vi "Send Test.vi"() -> ()   [LabVIEW 2009]
uses:
  UDP Lib/UDP Network Location.ctl
  Support Files/Address.ctl
  <vilib>/Platform/TimedLoop/XDataNode/XDataNode.xnode
  <vilib>/Platform/TimedLoop/XDataNode/loadlvalarms.vi
  <vilib>/Platform/TimedLoop/XDataNode/timing_clust.ctl
  <vilib>/Platform/TimedLoop/XDataNode/nitl_modes.ctl
  <vilib>/Platform/TimedLoop/XDataNode/wakeup.ctl
  <vilib>/Platform/TimedLoop/XDataNode/XDNodeRunTimeDep.lvlib
panel:
  out "Network Location":T1={"IP Address"="0.0.0.0", "Port"=0}
  out "Address Cluster":T2={"Subsystem Id"=90, "Node Id"=1, "Component Id"=1}
  out "Payload":string
  out "UDP Read Loop":bool=TRUE
  out "HB":bool
  in  "stop":bool
  in  "Destination Location":T1={"IP Address"="localhost", "Port"=3794}
  in  "Send":bool
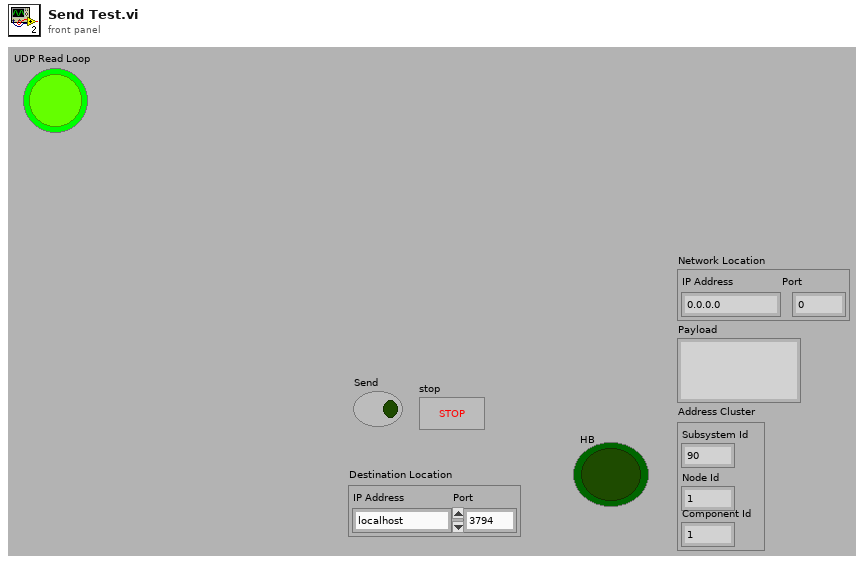
[diagram p1: front panel]
types:
  T1 = typedef "UDP Network Location.ctl" = cluster{"IP Address":string, "Port":u16}
  T2 = typedef "Address.ctl" = cluster{"Subsystem Id":u16, "Node Id":u8, "Component Id":u8}
  T3 = typedef "UDP Base.ctl" = cluster{"UDP Session":refnum<k16>, "UDP Socket Params":T4}
  T4 = typedef "UDP Socket Params.ctl" = cluster{"Local Port":u16, "Read Timeout":i32, "Write Timeout":i32}
  T5 = typedef "XDNodeRunTimeDep.lvlib/timing_clust.ctl" = cluster{"Expected End [f-1]":u64, "Actual End [f-1]":u64, "Finished Late? [f-1]":bool, "Expected End [i-1]":u64, "Actual End [i-1]":u64, "Finished Late? [i-1]":bool, "Expected Start [i]":u64, "Actual Start [i]":u64, "Expected Start [f]":u64, "Actual Start [f]":u64, "Source Name":string, "Structure Name":string, "Period":i64, "Deadline":i64, "Offset":i64, "Start":i64, "Priority":i32, "Timeout":i32, "Mode":T6, "Wakeup Reason":T7, "Error":errorcluster, "Source Type":string, "Secondary Source Type":string, "Global End Time":u64, "Global Start Time":u64, "Frame Duration":u64, "Iteration Duration":u64, "Assigned CPU":i32, "I/O Scan Engine Mode":u32}
  T6 = typedef "XDNodeRunTimeDep.lvlib/nitl_modes.ctl" = enum32{"No Change", "Process missed periods, maintain original phase", "Discard missed periods, maintain original phase", "Process missed periods, ignore original phase", "Discard missed periods, ignore original phase"}
  T7 = typedef "XDNodeRunTimeDep.lvlib/wakeup.ctl" = enum32{"Normal", "Aborted", "Asynchronous wakeup", "Timing source error", "Timed loop error", "Timeout"}
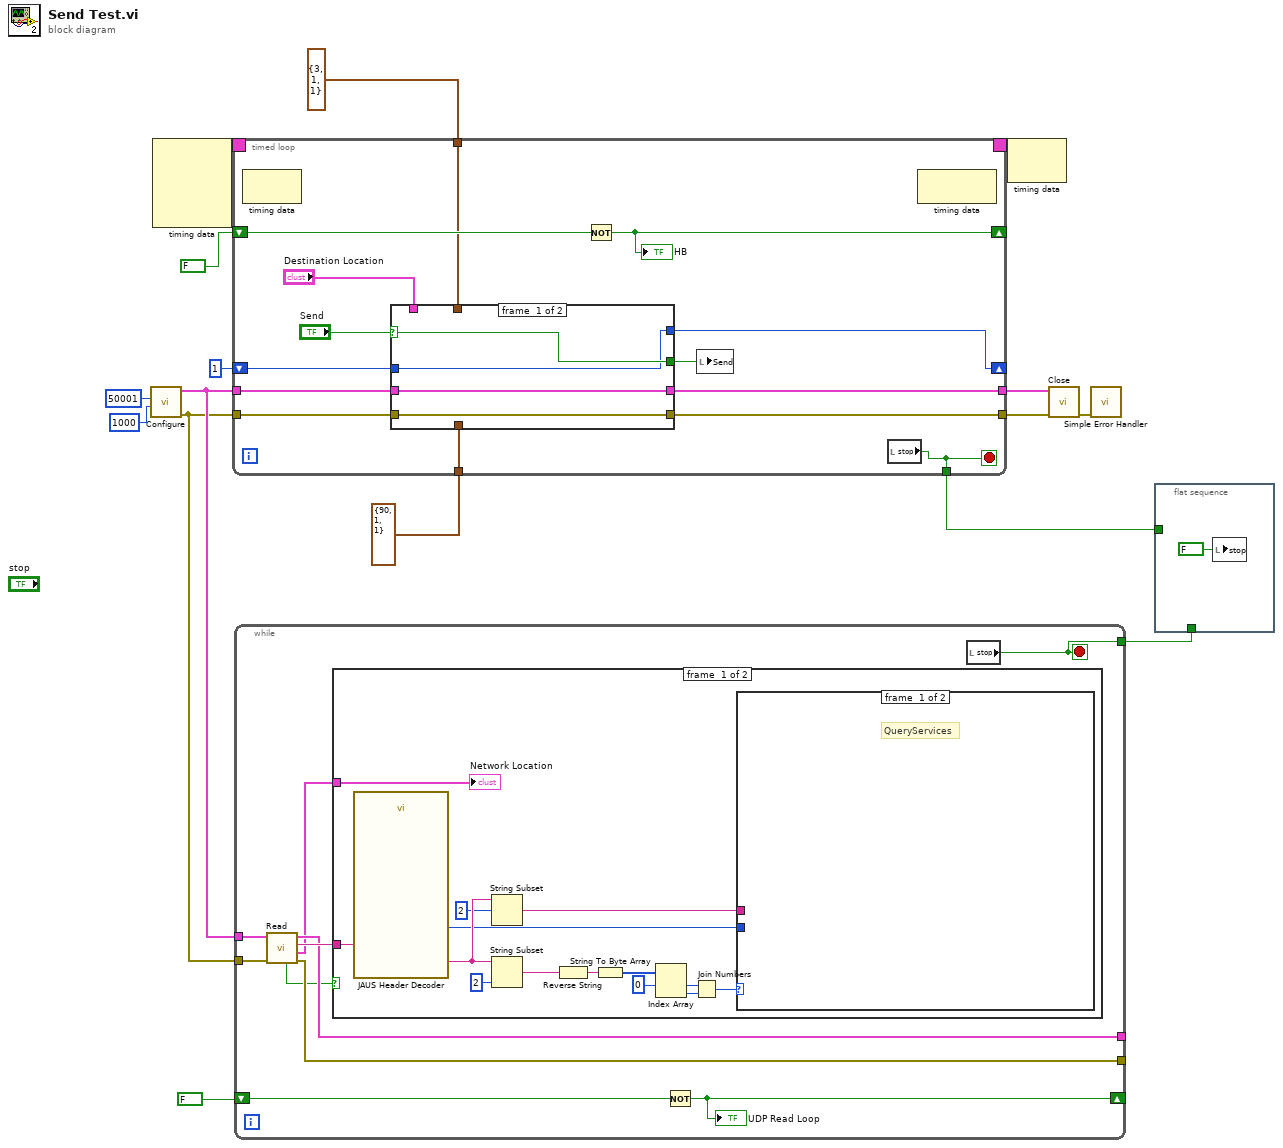
[diagram p0: block diagram]
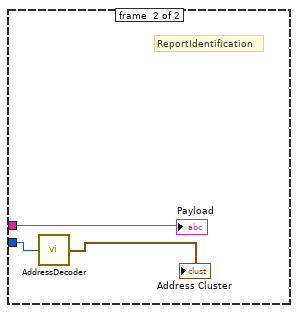
[diagram p2: hidden frame]
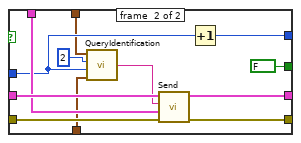
[diagram p4: hidden frame]
diagram:
  n1 = call "Configure.vi"("Read Timeout"=1000, "Local Port"=u16 50001) -> ("error out"=w1:errorcluster, "UDP Base out"=w2:T3)  [unwired: 8 in]
  n2 = node-c288() -> (w16:T5)  [unwired: 4 in]
  n3 = timed-loop {
    timing: w16 -> [_]
    timing-out: [_] -> w15
    tunnel: w2 -> [w28]
    tunnel: w1 -> [w27]
    shift-right: [w24] -> _
    shift-left: u16 1 ("Sequence Number (16 bits)") -> [w25]
    tunnel: [w23] -> w11
    tunnel: [w22] -> w10
    shift-right: [w20] -> _
    shift-left: FALSE -> [w21]
    tunnel: T2 {"Subsystem Id"=3, "Node Id"=1, "Component Id"=1} ("Source") -> [w19]
    tunnel: T2 {"Subsystem Id"=90, "Node Id"=1, "Component Id"=1} ("Destination") -> [w18]
    tunnel: [w17] -> w3
    stop <- w17 stop-if-true
    n4 = node-c288() -> ()  [unwired: 1 in, 1 out]
    n5 = case shown="True" "Send" {
      selector: "Send" -> [w36 _]
      tunnel: [w36 FALSE] -> w29
      tunnel: w28 -> [w34 w48]
      tunnel: w27 -> [w33 w47]
      tunnel: "Destination Location" -> [_ w46]
      tunnel: w25 -> [w35 w44]
      tunnel: [w35 w43] -> w24
      tunnel: [w34 w41] -> w23
      tunnel: [w33 w40] -> w22
      tunnel: w19 -> [_ w38]
      tunnel: w18 -> [_ w37]
      frame #0 {
      }
      frame #1 {
        n6 = call "QueryIdentification.vi"("Destination"=w37, "Sequence Number (16 bits)"=w44, "QueryType"=u8 2, "Source"=w38) -> ("Encoded JAUS Message"=w45:string)
        n7 = call "Send.vi"("error in (no error)"=w47, "Destination Location"=w46, "Send Data"=w45, "UDP Base in"=w48) -> ("error out"=w40:errorcluster, "UDP Base out"=w41:T3)  [unwired: 5 in, 1 out]
        n8 = Increment(x=w44) -> (x+1=w43:u16)
      }
    }
    n9 = Not(x=w21) -> (.not. x?=w20:bool)
    "HB" <- w20
    n10 = local write "Send"(w29) -> ()
    n11 = local read "stop"() -> (w17:bool)
    n12 = node-c288() -> ()  [unwired: 1 in, 1 out]
  }
  n13 = while {
    tunnel: w2 -> [w57]
    tunnel: w1 -> [w58]
    tunnel: [w55] -> _
    tunnel: [w54] -> _
    tunnel: [w49] -> w4
    shift-right: [w52] -> _
    shift-left: FALSE ("stop") -> [w53]
    stop <- w49 stop-if-true
    n14 = call "Read.vi"("error in (no error)"=w58, "UDP Base in"=w57) -> ("error out"=w54:errorcluster, "Network Location"=w50:T1, "Receive Data"=w56:string, "UDP Base out"=w55:T3, "Timeout"=w51:bool)  [unwired: 4 in, 1 out]
    n15 = case shown="False" w51 {
      tunnel: w56 -> [w61 _]
      tunnel: w50 -> [w59 _]
      frame #0 {
        n16 = call "JAUS Header Decoder.vi"("Encoded JAUS Message"=w61) -> ("Source ID (80-95)"=w60:u32, "Payload"=w64:string)  [unwired: 13 in, 12 out]
        n17 = String Subset(string=w64, offset (0)=2) -> (substring=w62:string)  [unwired: 1 in]
        n18 = String Subset(string=w64, length (rest)=2 ("length (rest)")) -> (substring=w65:string)  [unwired: 1 in]
        n19 = Reverse String(1:w65) -> (0:w68:string)
        n20 = String To Byte Array(string=w68) -> (unsigned byte array=w72:u8[])
        n21 = Index Array(array=w72, index #1=0 ("index")) -> (element #1=w70:u8, element #2=w69:u8)  [unwired: 1 in]
        n22 = Join Numbers(hi=w70, lo=w69) -> ((hi.lo)=w66:u16)
        n23 = case shown="4B00" w66 {
          tunnel: w62 -> [_ w75]
          tunnel: w60 -> [_ w74]
          frame #0 {
            # "QueryServices"
          }
          frame #1 {
            # "ReportIdentification"
            n24 = call "AddressDecoder.vi"("Address"=w74) -> ("Address Cluster"=→"Address Cluster":T2)
            "Payload" <- w75
          }
        }
        "Network Location" <- w59
      }
      frame #1 {
      }
    }
    n25 = Not(x=w53) -> (.not. x?=w52:bool)
    "UDP Read Loop" <- w52
    n26 = local read "stop"() -> (w49:bool)
  }
  n27 = node-c288(w15) -> ()  [unwired: 1 out]
  n28 = call "Close.vi"("error in (no error)"=w10, "Cluster of class private data"=w11) -> ("error out"=w9:errorcluster)  [unwired: 9 in]
  n29 = call <vilib>:"Simple Error Handler.vi"("error in (no error)"=w9) -> ()  [unwired: 4 in, 5 out]
  n30 = flat-sequence {
    tunnel: w4 -> [_]
    tunnel: w3 -> [_]
    frame #0 {
      n31 = local write "stop"(FALSE ("stop")) -> ()
    }
  }
